vi "MTCDT new test.vi"() -> ()   [LabVIEW 2024]
uses:
  MTCDT_radio_type.ctl
  Global 2.vi
panel:
  out "BT mac":string
  out "wifi mac":string
  in  "RadioType":T1=enum."L4N1"
  out "CMD line args":string[](array[string])
  in  "Save to log file (N)":bool
  in  "Loops":u32=1 min=1 step=1
  out "All Passed?":bool
  in  "VISA resource name":refnum<visa-resource-name>="COM5"
  out "error out":errorcluster
  in  "error in (no error)":errorcluster
  in  "Start":bool
  out "Test Log":string
  # "MTCDT test"
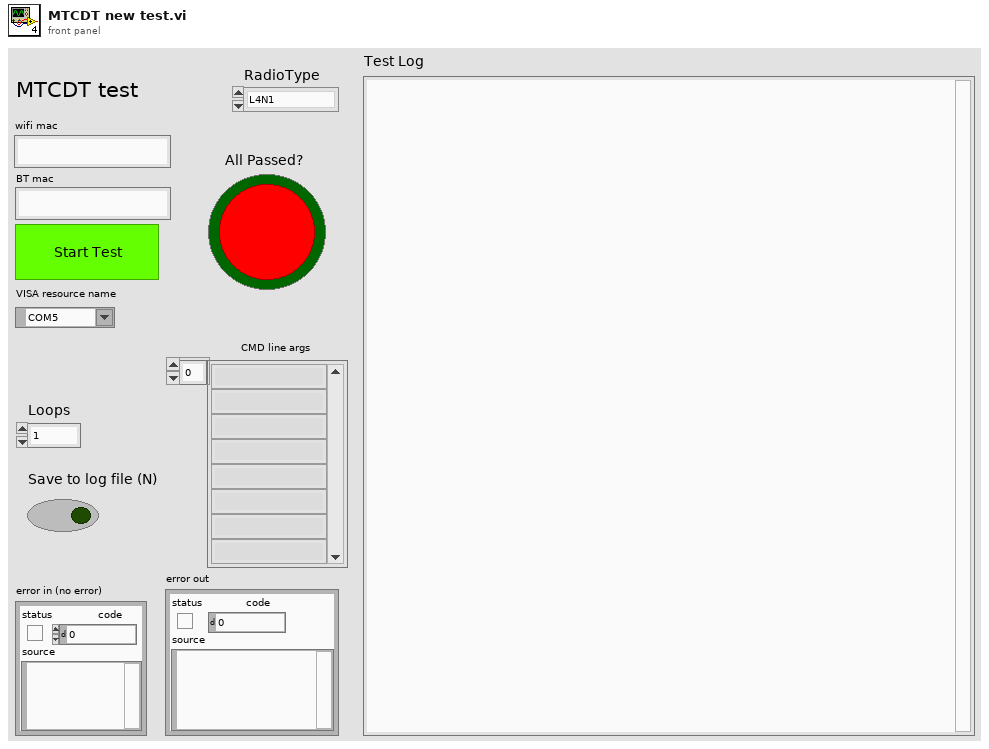
[diagram p1: front panel]
types:
  T1 = typedef "MTCDT_radio_type.ctl" = enum16{"LAT1", "H5", "LAT3", "LEU1", "L4E1", "L4N1", "LVW2", "LSB3", "LDC3", "LAP3", "L4G1", "L6G1"}
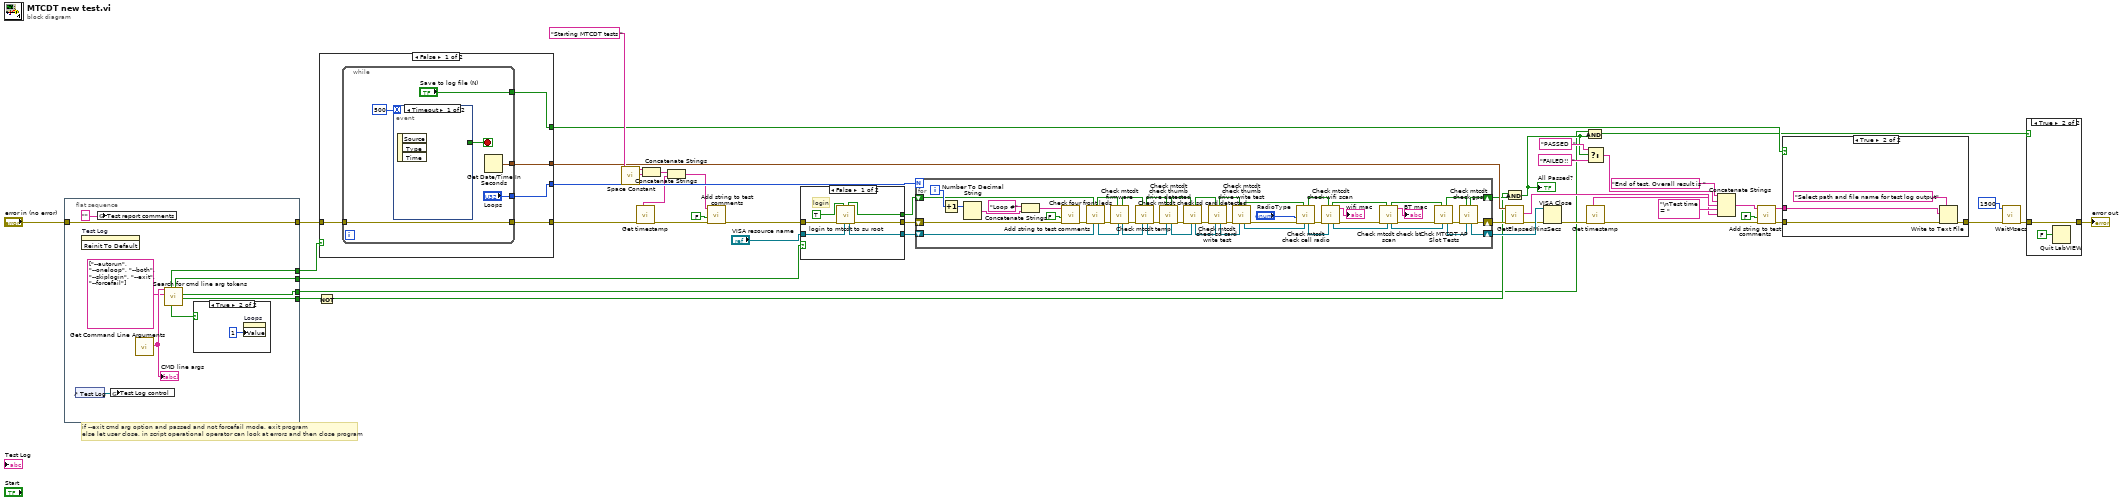
[diagram p0: block diagram]
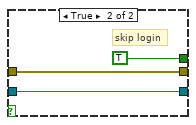
[diagram p3: hidden frame]
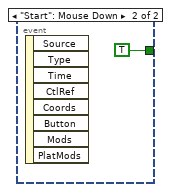
[diagram p4: hidden frame]
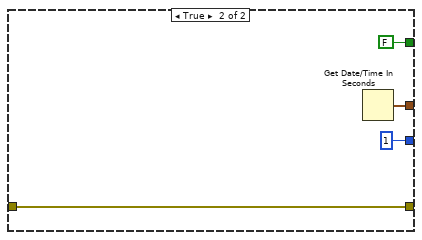
[diagram p5: hidden frame]
diagram:
  # "if --exit cmd arg option and passed and not forcefail mode, exit program\nelse let user close, in script operational operator can look at errors and then close program"
  n1 = flat-sequence {
    tunnel: [w56] -> w46
    tunnel: "error in (no error)" -> [w56]
    tunnel: [w48] -> w13
    tunnel: [w49] -> w12
    tunnel: [w50] -> w4
    tunnel: [w47] -> w8
    frame #0 {
      n2 = control-ref of="Test Log"() -> (w55:refnum<vi>)
      n3 = invoke on="Test Log" class="Str" method="Reinit To Default"() -> ()  [unwired: 3 in, 3 out]
      n4 = global write "Global 2.vi" "Test report comments"("" ("Test report comments")) -> ()
      n5 = global write "Global 2.vi" "Test Log control"(w55) -> ()
      n6 = call <vilib>:"Get Command Line Arguments.vi"() -> ("arguments"=w53:string[])  [unwired: 9 in, 2 out]
      "CMD line args" <- w53
      n7 = call "Search for cmd line arg tokens.vi"("look for tokens"=string[] ["--autorun", "--oneloop", "--both", "--skiplogin", "--exit", "--forcefail"], "table"=w53) -> ("[5]"=w47:bool, "[4]"=w50:bool, "[3]"=w49:bool, "[1]"=w51:bool, "[0]"=w48:bool)  [unwired: 2 in, 3 out]
      n8 = case shown="True" w51 {
        frame False {
        }
        frame True {
          n9 = property on="Loops" class="DigNum (strict)"("Value"=u32 1 ("Loops")) -> ()  [unwired: 2 in, 2 out]
        }
      }
    }
  }
  n10 = Not(x=w8) -> (.not. x?=w6:bool)
  n11 = case shown="False" w13 {
    tunnel: w46 -> [w62 w70]
    tunnel: [w61 u32 1 ("Loops")] -> w30
    tunnel: [w60 FALSE ("Save to log file (N)")] -> w28
    tunnel: [w59 w70] -> w26
    tunnel: [w58 w73] -> w16
    frame False {
      n12 = while {
        tunnel: [w67] -> w59
        tunnel: w62 -> [w67]
        tunnel: ["Loops"] -> w61
        tunnel: ["Save to log file (N)"] -> w60
        tunnel: [w64] -> w58
        stop <- w63 stop-if-true
        n13 = event shown="[0] Timeout" {
          selector: _ -> [_ _]
          dyn-events: _ -> [_ _]
          timeout: 500 -> [_ _]
          tunnel: [_ TRUE] -> w63
          event Timeout {
            n14 = event-data() -> ()  [unwired: 1 in, 3 out]
          }
          event "Start": Mouse Down {
            n15 = event-data() -> ()  [unwired: 1 in, 8 out]
          }
        }
        n16 = Get Date/Time In Seconds() -> (seconds since 1Jan1904=w64:timestamp)
      }
    }
    frame True {
      n17 = Get Date/Time In Seconds() -> (seconds since 1Jan1904=w73:timestamp)
    }
  }
  n18 = call <vilib>:"Space Constant.vi"() -> ("String"=w19:string)
  n19 = call "Get timestamp.vi"("error in (no error)"=w26) -> ("error out"=w25:errorcluster, "Date_time_for_filenames"=w24:string)  [unwired: 2 in, 7 out]
  n20 = Concatenate Strings("Starting MTCDT tests " ("Comments"), w19) -> (w2:string)
  n21 = Concatenate Strings(w2, w24) -> (w23:string)
  n22 = call "Add string to test comments.vi"("error in (no error)"=w25, "New Section (y)?"=FALSE, "Comments"=w23) -> ("error out"=w39:errorcluster)  [unwired: 7 in, 1 out]
  n23 = case shown="False" w12 {
    tunnel: [w79 w81] -> w44
    tunnel: "VISA resource name" -> [w78 w82]
    tunnel: [w77 TRUE ("Passed?")] -> w42
    tunnel: [w76 w82] -> w41
    tunnel: w39 -> [w74 w81]
    frame False {
      # "login"
      n24 = call "login to mtcdt to su root.vi"("VISA resource name"=w78, "Passed so far?"=TRUE, "error in (no error)"=w74) -> ("error out"=w79:errorcluster, "VISA resource name out"=w76:refnum<visa-resource-name>, "Passed?"=w77:bool)  [unwired: 4 in, 2 out]
    }
    frame True {
      # "skip login"
    }
  }
  n25 = for {
    N: w30 -> [_]
    shift-right: [w91] -> w18
    shift-left: w44 -> [w131]
    shift-right: [w89] -> w7
    shift-left: w42 -> [w84]
    shift-right: [w92] -> w32
    shift-left: w41 -> [w86]
    i -> [w130]
    n26 = Increment(x=w130) -> (x+1=w129:i32)
    n27 = Number To Decimal String(number=w129) -> (decimal integer string=w127:string)  [unwired: 1 in]
    n28 = Concatenate Strings("Loop #" ("string"), w127) -> (w126:string)
    n29 = call "Add string to test comments.vi"("error in (no error)"=w131, "New Section (y)?"=FALSE, "Comments"=w126) -> ("error out"=w88:errorcluster)  [unwired: 7 in, 1 out]
    n30 = call "Check four front leds.vi"("VISA resource name"=w86, "Passed so far"=w84, "error in (no error)"=w88) -> ("error out"=w87:errorcluster, "VISA Refnum out"=w85:refnum<visa-resource-name>, "Passed?"=w83:bool)  [unwired: 6 in]
    n31 = call "Check mtcdt firmware.vi"("VISA resource name"=w85, "Passed so far"=w83, "error in (no error)"=w87) -> ("error out"=w124:errorcluster, "VISA Refnum out"=w123:refnum<visa-resource-name>, "Passed?"=w122:bool)  [unwired: 4 in, 2 out]
    n32 = call "Check mtcdt temp.vi"("VISA resource name"=w123, "Passed so far"=w122, "error in (no error)"=w124) -> ("error out"=w121:errorcluster, "VISA Refnum out"=w120:refnum<visa-resource-name>, "Passed?"=w119:bool)  [unwired: 4 in, 2 out]
    n33 = call "Check mtcdt check thumb drive detected.vi"("VISA resource name"=w120, "Passed so far"=w119, "error in (no error)"=w121) -> ("error out"=w118:errorcluster, "VISA Refnum out"=w117:refnum<visa-resource-name>, "Passed?"=w116:bool)  [unwired: 4 in, 2 out]
    n34 = call "Check mtcdt check sd card detected.vi"("VISA resource name"=w117, "Passed so far"=w116, "error in (no error)"=w118) -> ("error out"=w115:errorcluster, "VISA Refnum out"=w113:refnum<visa-resource-name>, "Passed?"=w114:bool)  [unwired: 4 in, 2 out]
    n35 = call "Check mtcdt check sd card write test.vi"("VISA resource name"=w113, "Passed so far"=w114, "error in (no error)"=w115) -> ("error out"=w112:errorcluster, "VISA Refnum out"=w110:refnum<visa-resource-name>, "Passed?"=w111:bool)  [unwired: 4 in, 2 out]
    n36 = call "Check mtcdt check thumb drive write test.vi"("VISA resource name"=w110, "Passed so far"=w111, "error in (no error)"=w112) -> ("error out"=w98:errorcluster, "VISA Refnum out"=w100:refnum<visa-resource-name>, "Passed?"=w99:bool)  [unwired: 4 in, 2 out]
    n37 = call "Check mtcdt check cell radio.vi"("VISA resource name"=w100, "Passed so far"=w99, "error in (no error)"=w98, "RadioType"="RadioType") -> ("error out"=w108:errorcluster, "VISA Refnum out"=w107:refnum<visa-resource-name>, "Passed?"=w101:bool)  [unwired: 3 in, 2 out]
    n38 = call "Check mtcdt check wifi scan.vi"("VISA resource name"=w107, "Passed so far"=w101, "error in (no error)"=w108) -> ("error out"=w105:errorcluster, "wifi mac"=→"wifi mac":string, "VISA Refnum out"=w104:refnum<visa-resource-name>, "Passed?"=w103:bool)  [unwired: 5 in]
    n39 = call "Check mtcdt check bt scan.vi"("VISA resource name"=w104, "Passed so far"=w103, "error in (no error)"=w105) -> ("error out"=w97:errorcluster, "BT mac"=→"BT mac":string, "VISA Refnum out"=w94:refnum<visa-resource-name>, "Passed?"=w96:bool)  [unwired: 5 in]
    n40 = call "Chck MTCDT AP Slot Tests.vi"("VISA resource  inname"=w94, "Passed so far?"=w96, "error in (no error)"=w97) -> ("error out"=w95:errorcluster, "Visa resource name out"=w93:refnum<visa-resource-name>, "All Passed?"=w90:bool)  [unwired: 6 in]
    n41 = call "Check mtcdt check gps.vi"("VISA resource name"=w93, "Passed so far"=w90, "error in (no error)"=w95) -> ("error out"=w91:errorcluster, "VISA Refnum out"=w92:refnum<visa-resource-name>, "Passed?"=w89:bool)  [unwired: 5 in, 1 out]
  }
  n42 = And(x=w6, y=w7) -> (x .and. y?=w5:bool)
  "All Passed?" <- w5
  n43 = call "GetElapsedMinsSecs.vi"("error in (no error)"=w18, "Op Start Time"=w16) -> ("error out"=w17:errorcluster, "ElapsedTime"=w14:string)  [unwired: 6 in, 2 out]
  n44 = VISA Close(VISA resource name=w32, error in (no error)=w17) -> (error out=w22:errorcluster)
  n45 = And(x=w4, y=w5) -> (x .and. y?=w3:bool)
  n46 = Select(t="PASSED  ", s=w5, f="FAILED!!  ") -> (s? t:f=w35:string)
  n47 = call "Get timestamp.vi"("error in (no error)"=w22) -> ("error out"=w20:errorcluster, "Date_time_for_filenames"=w21:string)  [unwired: 2 in, 7 out]
  n48 = Concatenate Strings("End of test. Overall result is " ("string"), w35, w21, "\nTest time = " ("string"), w14) -> (w34:string)
  n49 = call "Add string to test comments.vi"("error in (no error)"=w20, "New Section (y)?"=FALSE, "Comments"=w34) -> ("error out"=w27:errorcluster, "concatenated string"=w29:string)  [unwired: 7 in]
  n50 = case shown="True" w28 {
    tunnel: w29 -> [_ w135]
    tunnel: w27 -> [w132 w136]
    tunnel: [w132 w133] -> w1
    frame False {
    }
    frame True {
      n51 = Write to Text File(prompt (Choose or enter file path)="Select path and file name for test log output", text=w135, error in=w136) -> (error out=w133:errorcluster)  [unwired: 1 in, 2 out]
    }
  }
  n52 = call "WaitMsecs.vi"("error in (no error)"=w1, "Wait Msecs"=u32 1500) -> ("error out"=w10:errorcluster)  [unwired: 9 in]
  n53 = case shown="True" w3 {
    tunnel: [w137 w139] -> w11
    tunnel: w10 -> [w137 w139]
    frame False {
    }
    frame True {
      n54 = Quit LabVIEW(quit? (T)=FALSE) -> ()
    }
  }
  "error out" <- w11
